vi "Set Property.vi"(8 "error in (no error)":errorcluster, 9 "Value":dbl, 10 "Property":string, 11 "ToneCloud in":refnum<class "Tone Cloud.lvclass">) -> (0 "error out":errorcluster, 3 "ToneCloud out":refnum<class "Tone Cloud.lvclass">)   [LabVIEW 2020, in "Tone Cloud.lvclass"]
uses:
  Tone Cloud.lvclass
  Tone Cloud.lvclass/Tone Cloud.ctl
  <vilib>/regexp/Match Regular Expression.xnode
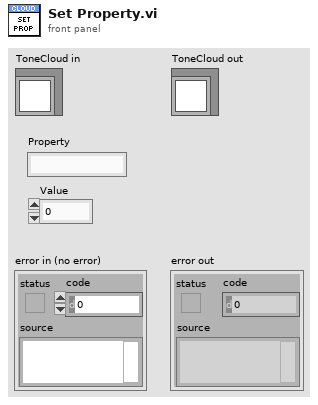
[diagram p1: front panel]
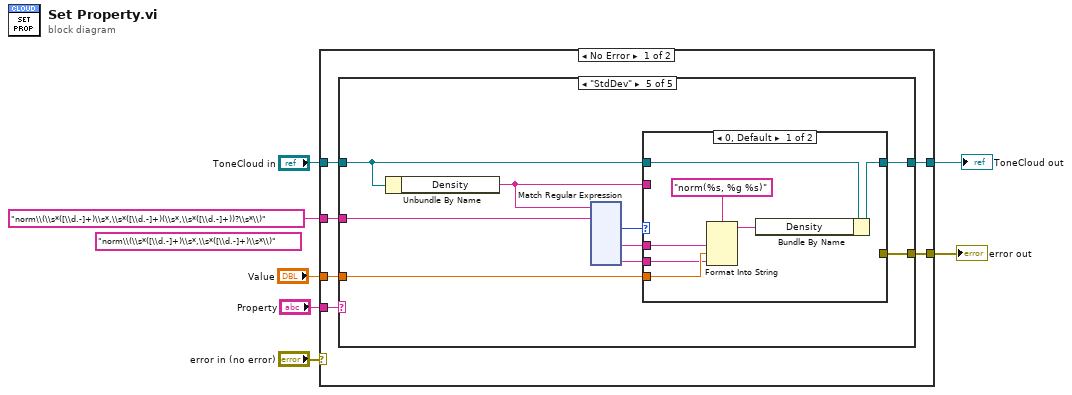
[diagram p0: block diagram]
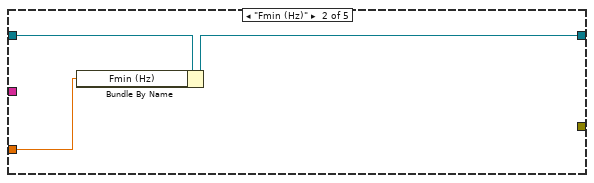
[diagram p3: hidden frame]
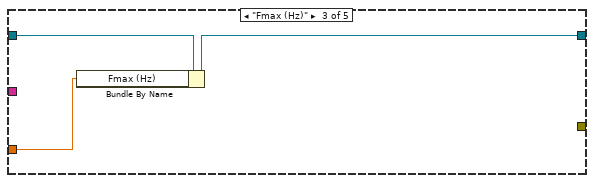
[diagram p4: hidden frame]
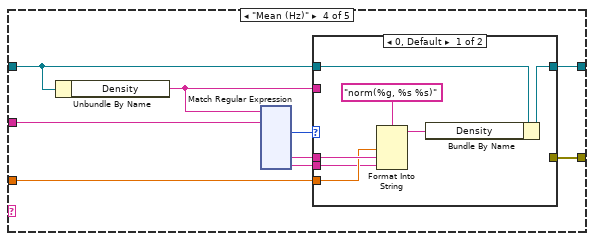
[diagram p5: hidden frame]
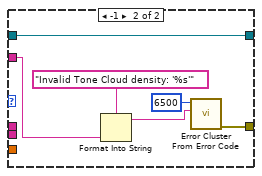
[diagram p6: hidden frame]
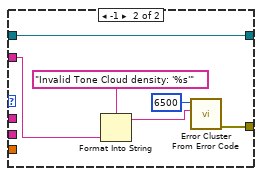
[diagram p7: hidden frame]
diagram:
  (unwired) "norm\\(\\s*([\\d.-]+)\\s*,\\s*([\\d.-]+)\\s*\\)" ("String")
  n1 = case shown="No Error" "error in (no error)" {
    selector: "error in (no error)" -> [_ w301]
    tunnel: [w9 w301] -> w5
    tunnel: "Property" -> [w13 _]
    tunnel: "ToneCloud in" -> [w12 w302]
    tunnel: "Value" -> [w11 _]
    tunnel: [w10 w302] -> w6
    tunnel: "norm\\(\\s*([\\d.-]+)\\s*,\\s*([\\d.-]+)(\\s*,\\s*([\\d.-]+))?\\s*\\)" ("String") -> [w8 _]
    frame No Error {
      n2 = case shown="\"StdDev\"" w13 {
        tunnel: w12 -> [w14 w17 w20 w29 w169]
        tunnel: w11 -> [_ w16 w19 w25 w166]
        tunnel: [w14 w15 w18 w27 w167] -> w10
        tunnel: [_ _ _ w24 w165] -> w9
        tunnel: w8 -> [_ _ _ w22 w162]
        frame "", Default {
        }
        frame "Fmin (Hz)" {
          n3 = Bundle By Name(cluster=w17, "Fmin (Hz)"=w16) -> (w15:refnum<class "Tone Cloud.lvclass">)
        }
        frame "Fmax (Hz)" {
          n4 = Bundle By Name(cluster=w20, "Fmax (Hz)"=w19) -> (w18:refnum<class "Tone Cloud.lvclass">)
        }
        frame "Mean (Hz)" {
          n5 = Unbundle By Name(w29) -> ("Density"=w23:string)
          n6 = xnode "Match Regular Expression"("input string"=w23, "regular expression"=w22) -> ("offset past match"=w28:i32, "submatch 2"=w26:string, "submatch 3"=w21:string)  [unwired: 4 in, 5 out]
          n7 = case shown="0, Default" w28 {
            tunnel: w29 -> [w36 w42]
            tunnel: [w35 w42] -> w27
            tunnel: w26 -> [w32 _]
            tunnel: w25 -> [w31 _]
            tunnel: [_ w40] -> w24
            tunnel: w23 -> [_ w38]
            tunnel: w21 -> [w30 _]
            frame 0, Default {
              n8 = Format Into String(format string="norm(%g, %s %s)", w31, w32, w30) -> (resulting string=w34:string)  [unwired: 2 in, 1 out]
              n9 = Bundle By Name(cluster=w36, "Density"=w34) -> (w35:refnum<class "Tone Cloud.lvclass">)
            }
            frame -1 {
              n10 = Format Into String(format string="Invalid Tone Cloud density: '%s'", w38) -> (resulting string=w37:string)  [unwired: 2 in, 1 out]
              n11 = call <vilib>:"Error Cluster From Error Code.vi"("error message (\"\")"=w37, "error code (0)"=6500) -> ("error out"=w40:errorcluster)  [unwired: 7 in]
            }
          }
        }
        frame "StdDev" {
          n12 = Unbundle By Name(w169) -> ("Density"=w164:string)
          n13 = xnode "Match Regular Expression"("input string"=w164, "regular expression"=w162) -> ("offset past match"=w168:i32, "submatch 1"=w163:string, "submatch 3"=w161:string)  [unwired: 4 in, 5 out]
          n14 = case shown="0, Default" w168 {
            tunnel: w169 -> [w176 w182]
            tunnel: [w175 w182] -> w167
            tunnel: w166 -> [w172 _]
            tunnel: [_ w180] -> w165
            tunnel: w164 -> [_ w178]
            tunnel: w163 -> [w171 _]
            tunnel: w161 -> [w170 _]
            frame 0, Default {
              n15 = Format Into String(format string="norm(%s, %g %s)", w171, w172, w170) -> (resulting string=w174:string)  [unwired: 2 in, 1 out]
              n16 = Bundle By Name(cluster=w176, "Density"=w174) -> (w175:refnum<class "Tone Cloud.lvclass">)
            }
            frame -1 {
              n17 = Format Into String(format string="Invalid Tone Cloud density: '%s'", w178) -> (resulting string=w177:string)  [unwired: 2 in, 1 out]
              n18 = call <vilib>:"Error Cluster From Error Code.vi"("error message (\"\")"=w177, "error code (0)"=6500) -> ("error out"=w180:errorcluster)  [unwired: 7 in]
            }
          }
        }
      }
    }
    frame Error {
    }
  }
  "error out" <- w5
  "ToneCloud out" <- w6
